vi "PolyVI.vi"   [LabVIEW 2017]
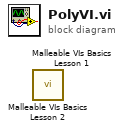
[diagram p0: block diagram]
diagram:
  n1 = call "Malleable VIs Basics Lesson 2.vi"() -> ()  [unwired: 11 in, 1 out]
  n2 = call "Malleable VIs Basics Lesson 1.vi"() -> ()  [unwired: 11 in, 1 out]
